vi "Polar 2 Cartisian, Plotting하기 위한 Vi.vi"(7 "X":dbl[][](array[numeric])) -> (0 "theta":dbl[](array[numeric]), 1 "r":dbl[](array[numeric]), 2 "y":dbl[](array[numeric]), 3 "x":dbl[](array[numeric]))   [LabVIEW 2016]
uses:
  <vilib>/imath/engines/lvmath2/RunTimeEngine/Managers/WorkSpace/UID Generator.vi
  <vilib>/imath/engines/lvmath2/RunTimeEngine/IndexRead/NIMS M($,S).vi
  <instcachedir>/0/NIMS M($,S)_3E5749BBB62E49528D4765A77F1F6D98.lvgen/NIMS M($,S)_3E5749BBB62E49528D4765A77F1F6D98_000.vi
  <vilib>/imath/engines/lvmath2/RunTimeEngine/RunTimeType/NIMS_RunTimeType_From StrictType (excl LVString).vi
  <instcachedir>/0/NIMS_RunTimeType_From StrictType (excl LVString)_BBF44FB49F834B71AF7A14CCEDF8BECD.lvgen/NIMS_RunTimeType_From StrictType (excl LVString)_BBF44FB49F834B71AF7A14CCEDF8BECD_000.vi
  <vilib>/imathl/engines/lvmath/Functions/Error Handling/Create Error.vi
  <vilib>/imath/engines/lvmath2/RunTimeEngine/LocalVariableDefStatement/MC_LocalVariableDefStatement_Display.vi
  <vilib>/imath/engines/lvmath2/RunTimeEngine/ArithmeticOperatorToken/NIMS_ArithmeticOperator_times.vi
  <instcachedir>/0/NIMS_ArithmeticOperator_times_953B34F74CAC448FB707D816A29CC5F0.lvgen/NIMS_ArithmeticOperator_times_953B34F74CAC448FB707D816A29CC5F0_000.vi
  <vilib>/imath/engines/lvmath2/RunTimeEngine/Managers/SymbolTable/Clear UID.vi
  <vilib>/imath/engines/lvmath2/RunTimeEngine/NodeEndStatement/NIMS_NodeEndStatement_Output.vi
  <instcachedir>/0/NIMS_NodeEndStatement_Output_53EC0D466D134D7ABD903AC30B43404B.lvgen/NIMS_NodeEndStatement_Output_53EC0D466D134D7ABD903AC30B43404B_005.vi
  <vilib>/imath/engines/lvmath2/RunTimeEngine/ErrorHandling/NIMS_Finalize Error.vi
  <vilib>/imath/engines/lvmath2/RunTimeEngine/Managers/SymbolTable/NIMS_WorkSpace.lvlib
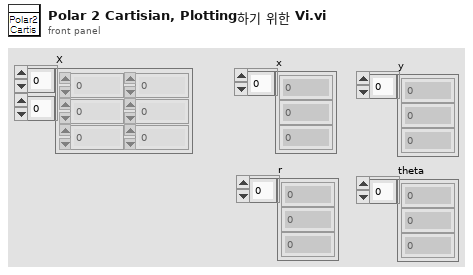
[diagram p1: front panel]
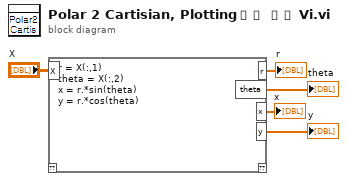
[diagram p0: block diagram]
diagram:
  n1 = mathscript code="r = X(:,1)\ntheta = X(:,2)\nx = r.*sin(theta)\ny = r.*cos(theta)"("X"="X") -> ("r"=→"r":dbl[], "theta"=→"theta":dbl[], "x"=→"x":dbl[], "y"=→"y":dbl[])  [unwired: 1 in, 1 out]
